vi "main.vi"() -> ()   [LabVIEW 2016]
uses:
  LibB/Options.ctl
  LibA/LibA.lvlib
  LibB/LibB.lvlib
panel:
  out "output":dbl
  in  "input":dbl
  out "Options":T1
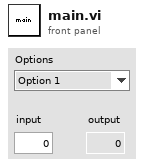
[diagram p1: front panel]
types:
  T1 = typedef "LibB.lvlib/Options.ctl" = enum16{"Option 1", "Option 2"}
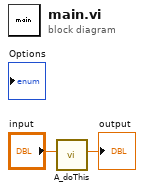
[diagram p0: block diagram]
diagram:
  n1 = call "A_doThis.vi"("input"="input") -> ("output"=→"output":dbl)  [unwired: 10 in]
